vi "parse_i64_scalar.vi"(4 "error in":errorcluster, 6 "type":i64, 7 "msg in":string) -> (0 "error out":errorcluster, 2 "number":i64, 3 "msg out":string)   [LabVIEW 2015]
doc: "Parses out a 64bit integer from msg in. The remaining string is returned in msg out."
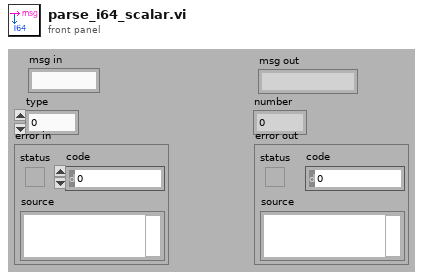
[diagram p1: front panel]
types:
  T1 = enum16{"big-endian, network order", "native, host order", "little-endian"}
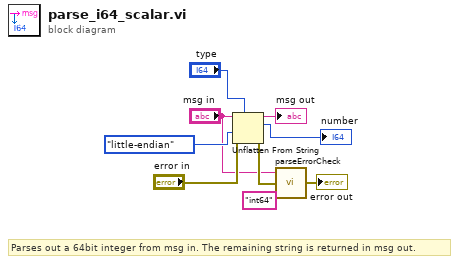
[diagram p0: block diagram]
diagram:
  # "Parses out a 64bit integer from msg in. The remaining string is returned in msg out."
  n1 = Unflatten From String(type="type", binary string="msg in", byte order (0:big-endian, network order)=T1."little-endian", error in (no error)="error in") -> (rest of the binary string=→"msg out":string, value=→"number":i64, error out=w5:errorcluster)  [unwired: 1 in]
  n2 = call "parseErrorCheck.vi"("type"="int64", "error in"=w5, "msg read"="msg in") -> ("error out"=→"error out":errorcluster)
